vi "POWER SUPPLY.vi"() -> ()   [LabVIEW 2017]
uses:
  <instrlib>/Keysight E36300 Series/Keysight E36300 Series.lvlib
panel:
  in  "Channel (1)":string="1"
  in  "Voltage Level (1 V)":dbl=1.0
  in  "VISA resource name":refnum<visa-resource-name>
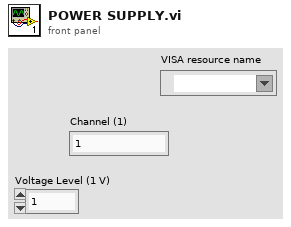
[diagram p1: front panel]
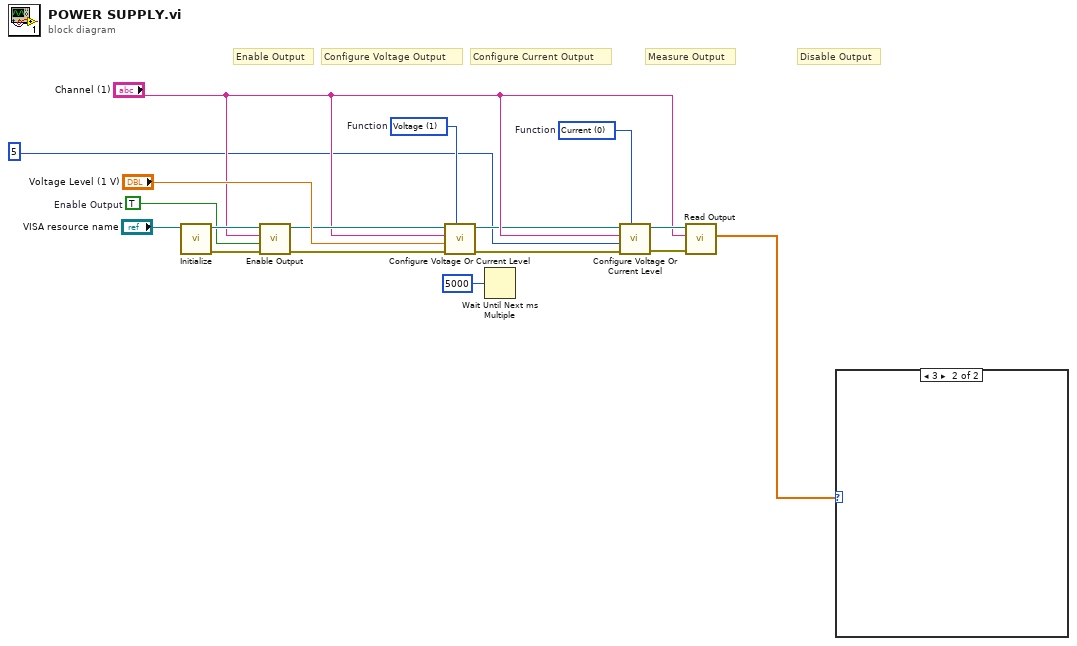
[diagram p0: block diagram]
diagram:
  w7 = 0 items=["Current", "Voltage"]  # Function
  w8 = 1 items=["Current", "Voltage"]  # Function
  w12 = TRUE  # Enable Output
  # "Disable Output"
  # "Configure Current Output"
  # "Configure Voltage Output"
  # "Measure Output"
  # "Enable Output"
  n1 = call <instrlib>:"Initialize.vi"("VISA resource name"="VISA resource name") -> ("error out"=w14:errorcluster, "VISA resource name out"=w15:refnum<visa-resource-name>)  [unwired: 9 in]
  n2 = call <instrlib>:"Enable Output.vi"("error in (no error)"=w14, "Enable Output (F: Disable)"=w12, "Channel (1)"="Channel (1)", "VISA resource name"=w15) -> ("error out"=w11:errorcluster, "VISA resource name out"=w13:refnum<visa-resource-name>)  [unwired: 6 in]
  n3 = call <instrlib>:"Configure Voltage Or Current Level.vi"("Function (0 : Current)"=w8, "error in (no error)"=w11, "Voltage Or Current Level (1)"="Voltage Level (1 V)", "Channel (1)"="Channel (1)", "VISA resource name"=w13) -> ("error out"=w5:errorcluster, "VISA resource name out"=w4:refnum<visa-resource-name>)  [unwired: 5 in]
  n4 = Wait Until Next ms Multiple(millisecond multiple=u32 5000) -> ()  [unwired: 1 out]
  n5 = call <instrlib>:"Configure Voltage Or Current Level.vi"("Function (0 : Current)"=w7, "error in (no error)"=w5, "Voltage Or Current Level (1)"=5, "Channel (1)"="Channel (1)", "VISA resource name"=w4) -> ("error out"=w6:errorcluster, "VISA resource name out"=w10:refnum<visa-resource-name>)  [unwired: 5 in]
  n6 = call <instrlib>:"Read Output.vi"("error in (no error)"=w6, "Channel (1)"="Channel (1)", "VISA resource name"=w10) -> ("Actual Voltage Level (V)"=w1:dbl[])  [unwired: 5 in, 3 out]
  n7 = case shown="3" w1 {
    frame 6 {
    }
    frame 3 {
    }
  }
